vi "Queue Access FGV.vi"(1 "FGV State Command":T1, 3 "error in (no error)":errorcluster) -> (7 "Queue out":refnum<queue>, 10 "error out":errorcluster)   [LabVIEW 2020]
uses:
  Controls/FGV State Command.ctl
  Controls/Message Data.ctl
  Controls/State Command.ctl
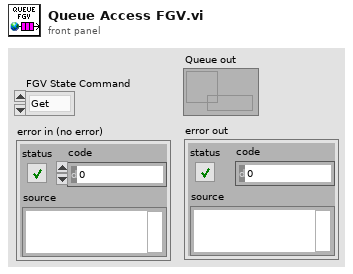
[diagram p1: front panel]
types:
  T1 = typedef "FGV State Command.ctl" = enum16{"Get", "Initialize", "Release"}
  T2 = typedef "Message Data.ctl" = cluster{"State Command":T3, "Data":variant}
  T3 = typedef "State Command.ctl" = enum16{"Display Message", "Stop"}
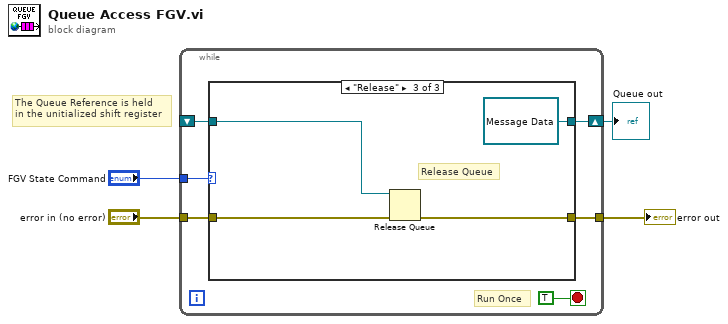
[diagram p0: block diagram]
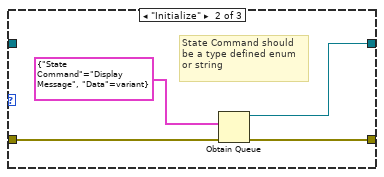
[diagram p3: hidden frame]
diagram:
  # "The Queue Reference is held\nin the unitialized shift register"
  n1 = while {
    tunnel: "FGV State Command" -> [w10]
    shift-right: [w8] -> w1
    shift-left: _ -> [w7]
    tunnel: [w6] -> w2
    tunnel: "error in (no error)" -> [w5]
    stop <- TRUE stop-if-true
    # "Run Once"
    n2 = case shown="\"Release\"" w10 {
      tunnel: [w12 w16 refnum<queue> refnum ("queue out")] -> w8
      tunnel: w7 -> [w12 _ w18]
      tunnel: [w11 w15 w19] -> w6
      tunnel: w5 -> [w11 w14 w20]
      frame "Get", Default {
      }
      frame "Initialize" {
        # "State Command should\nbe a type defined enum\nor string"
        n3 = Obtain Queue(element data type=T2 {"State Command"=enum."Display Message", "Data"=variant} ("Message Data"), error in (no error)=w14) -> (queue out=w16:refnum<queue>, error out=w15:errorcluster)  [unwired: 3 in, 1 out]
      }
      frame "Release" {
        # "Release Queue"
        n4 = Release Queue(queue=w18, error in (no error)=w20) -> (error out=w19:errorcluster)  [unwired: 1 in, 2 out]
      }
    }
  }
  "error out" <- w2
  "Queue out" <- w1
